vi "Deadband.vi"(11 "upper limit":dbl) -> (1 "in deband":bool, 3 "Numeric":dbl)   [LabVIEW 2020]
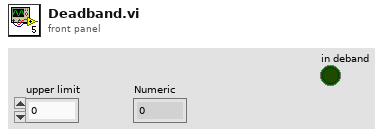
[diagram p1: front panel]
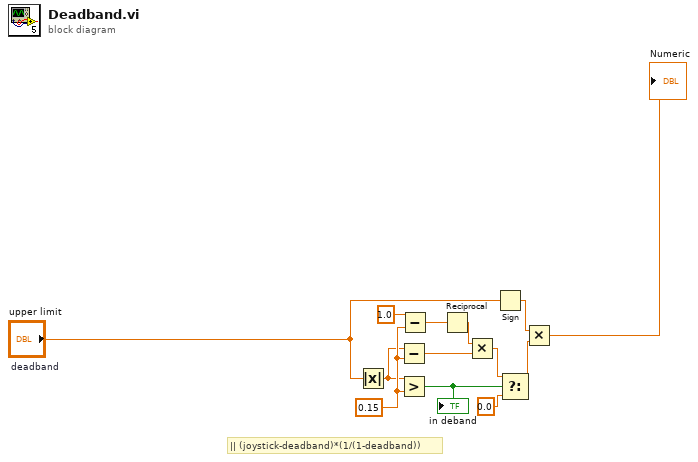
[diagram p0: block diagram]
diagram:
  w7 = 0.15  # deadband
  # "|| (joystick-deadband)*(1/(1-deadband))"
  n1 = Absolute Value(x="upper limit") -> (abs(x)=w3:dbl)
  n2 = Subtract(x=w3, y=w7) -> (x-y=w4:dbl)
  n3 = Greater?(x=w3, y=w7) -> (0:w2:bool)
  "in deband" <- w2
  n4 = Subtract(x=1.0 ("f"), y=w7) -> (x-y=w8:dbl)
  n5 = Reciprocal(x=w8) -> (1/x=w5:dbl)
  n6 = Multiply(x=w5, y=w4) -> (x*y=w9:dbl)
  n7 = Sign(1:"upper limit") -> (0:w11:dbl)
  n8 = Select(t=w9, s=w2, f=0.0) -> (s? t:f=w12:dbl)
  n9 = Multiply(x=w11, y=w12) -> (x*y=→"Numeric":dbl)
